vi "#EVENT Main.vi"() -> ()   [LabVIEW 2013]
panel:
  in  "BOOLEAN":bool
  out "COLD STORAGE LOCATIONS":string
  out "LOW MOISTURE":bool
  out "INTERMEDIATE MOISTURE":bool
  out "HIGH MOISTURE":bool
  out "MOISTURE LEVEL(ppm)":dbl
  out "pH VALUE":dbl
  out "SUGGESTED CROP":string
  out "Alert":bool
  out "POSITION":string
  out "Current Latitude [deg]":string
  out "Current Longitude [deg]":string
  in  "USER EMAIL Id":string="pankaj7897@outlook.com"
  out "CURRENT FARM STATUS":T1(plugin-control)
  out "WEATHER FORECAST":T2(array[cluster])
  # "SOIL ANALYSIS REPORT"
  # "SECURITY REPORT"
  # "MOISTURE READINGS"
  # "COLD STORAGE HOUSES NEAR YOU"
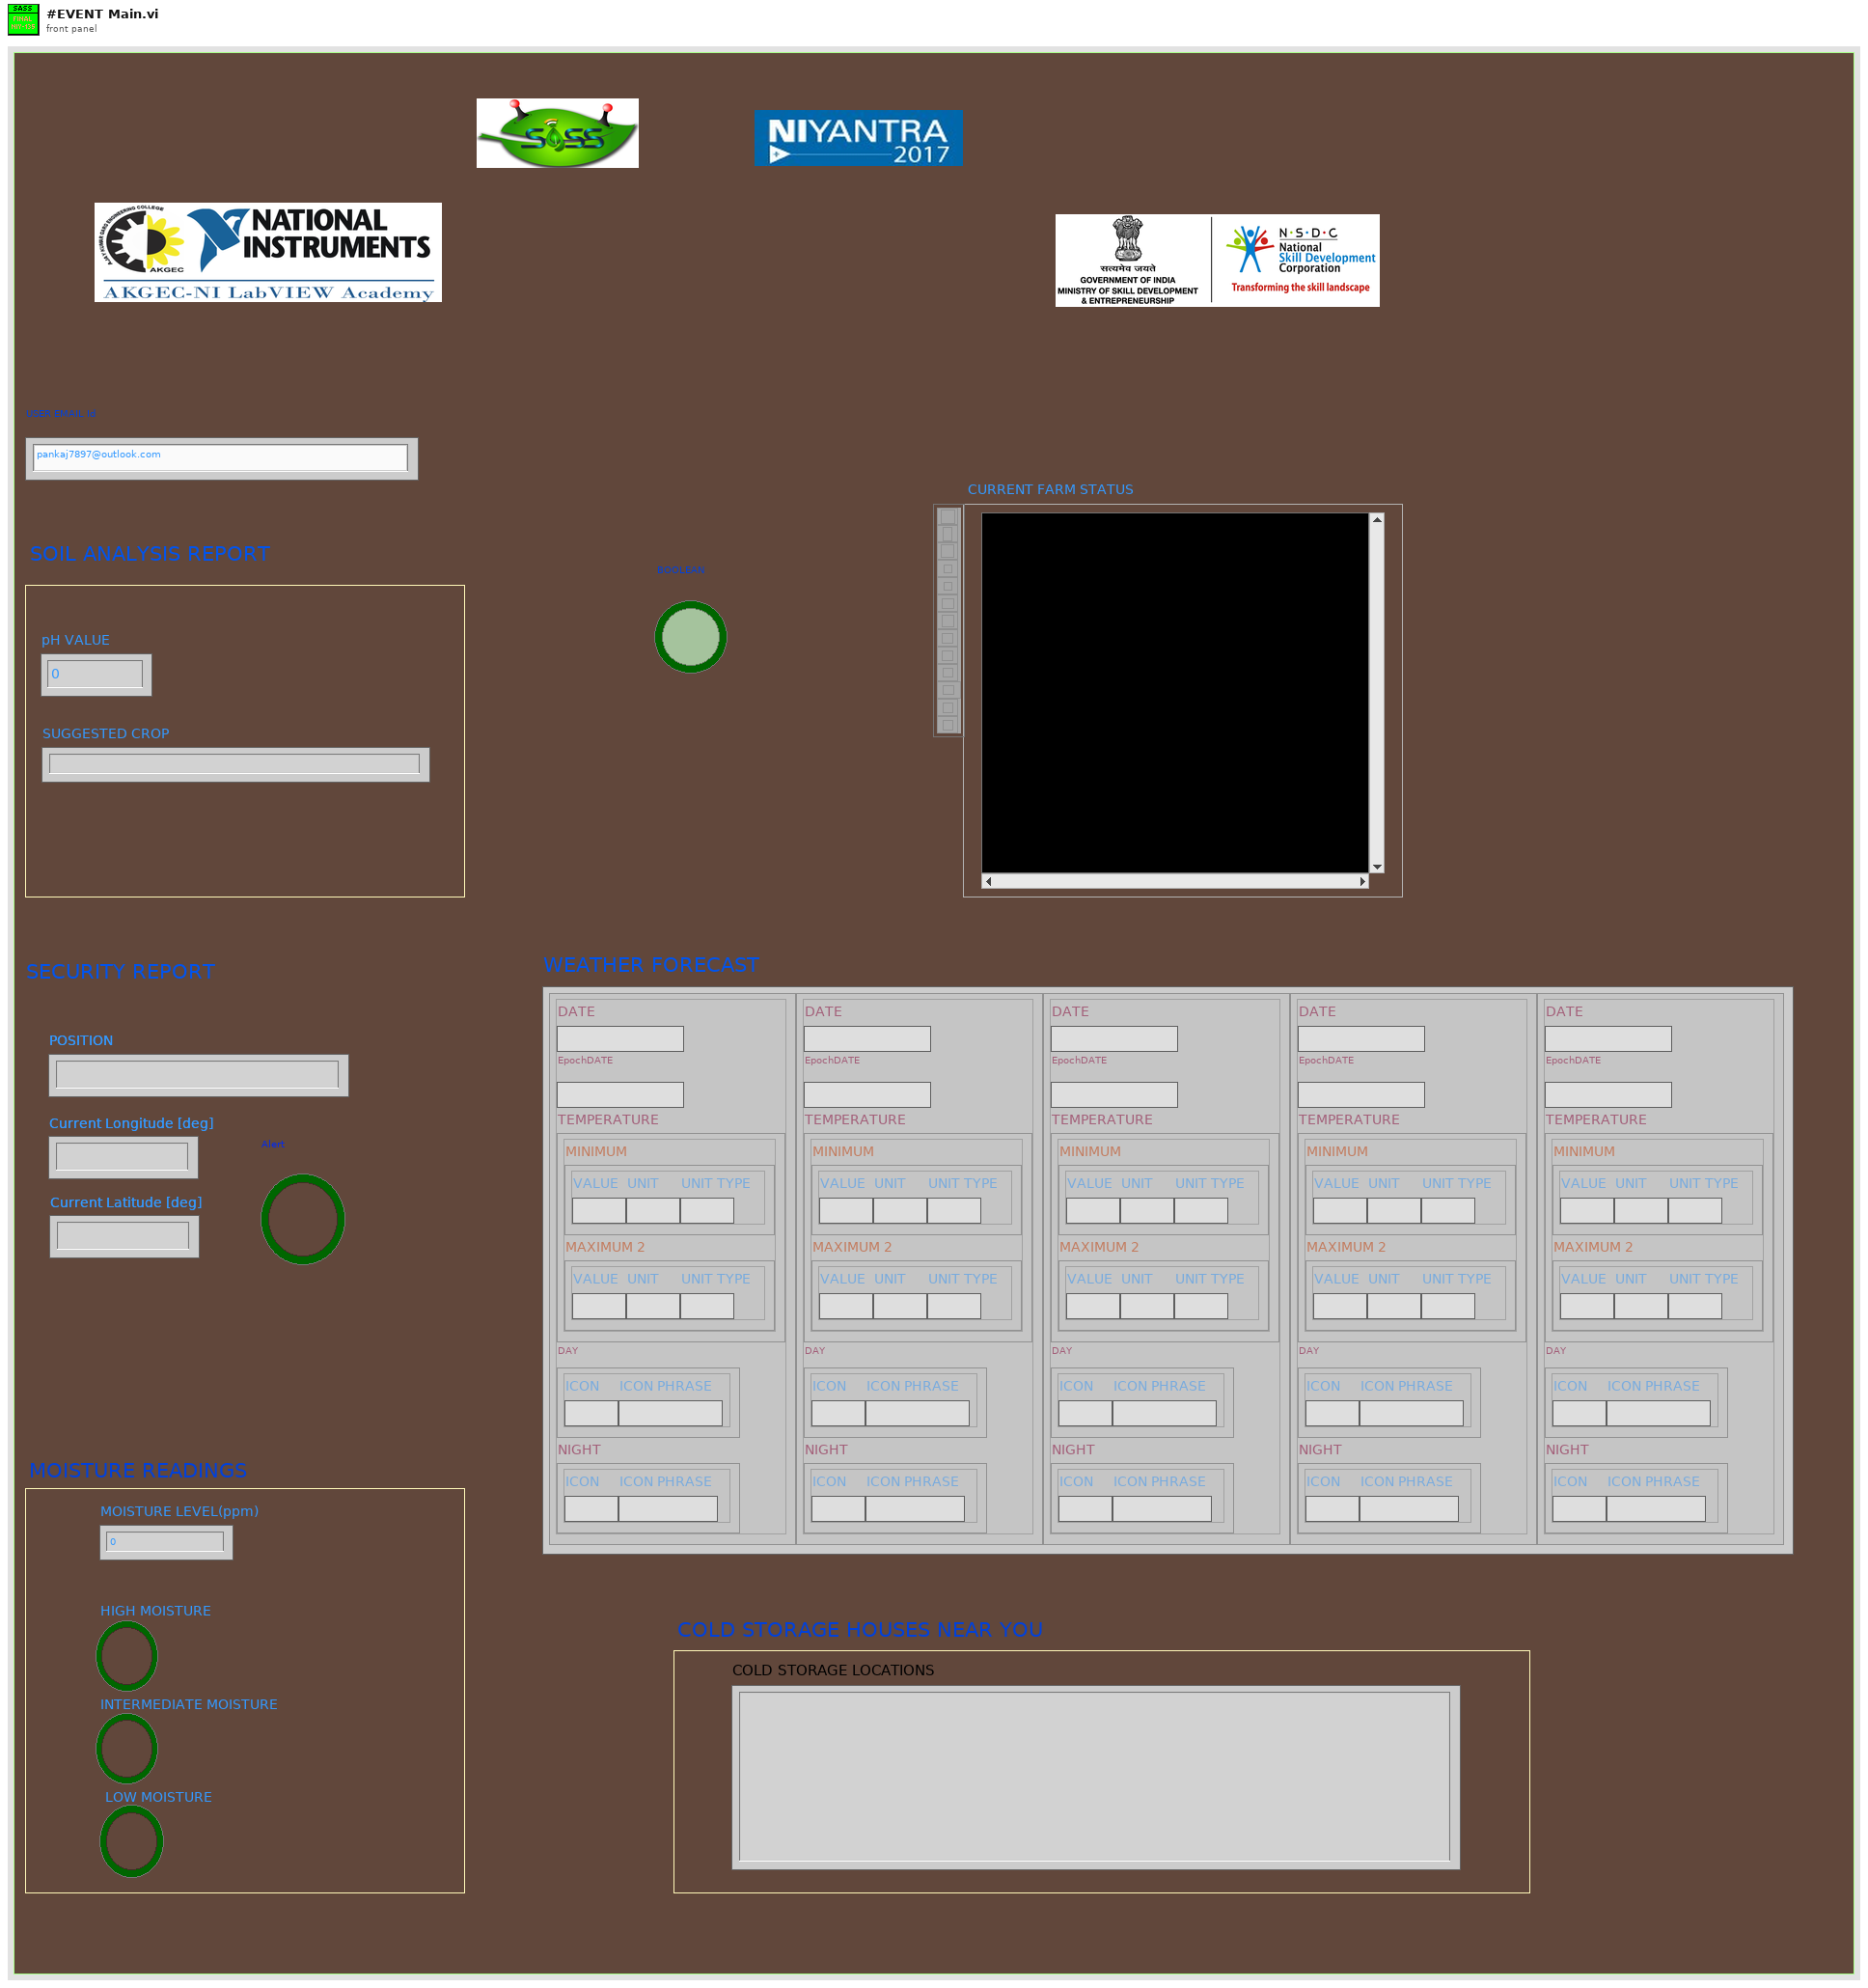
[diagram p1: front panel]
types:
  T1 = typedef "IMAQ Image.ctl" = refnum<image>
  T2 = cluster{"DATE":string, "EpochDATE":string, "TEMPERATURE":cluster{"MINIMUM":cluster{"VALUE":string, "UNIT":string, "UNIT TYPE":string}, "MAXIMUM 2":cluster{"VALUE":string, "UNIT":string, "UNIT TYPE":string}}, "DAY ":cluster{"ICON":string, "ICON PHRASE":string}, "NIGHT":cluster{"ICON":string, "ICON PHRASE":string}}[]
  T3 = cluster{"DATE":string, "EpochDATE":string, "TEMPERATURE":cluster{"MINIMUM":cluster{"VALUE":string, "UNIT":string, "UNIT TYPE 3":string}, "MAXIMUM 2":cluster{"VALUE":string, "UNIT":string, "UNIT TYPE":string}}, "DAY ":cluster{"ICON":string, "ICON PHRASE":string}, "NIGHT":cluster{"ICON":string, "ICON PHRASE":string}}[]
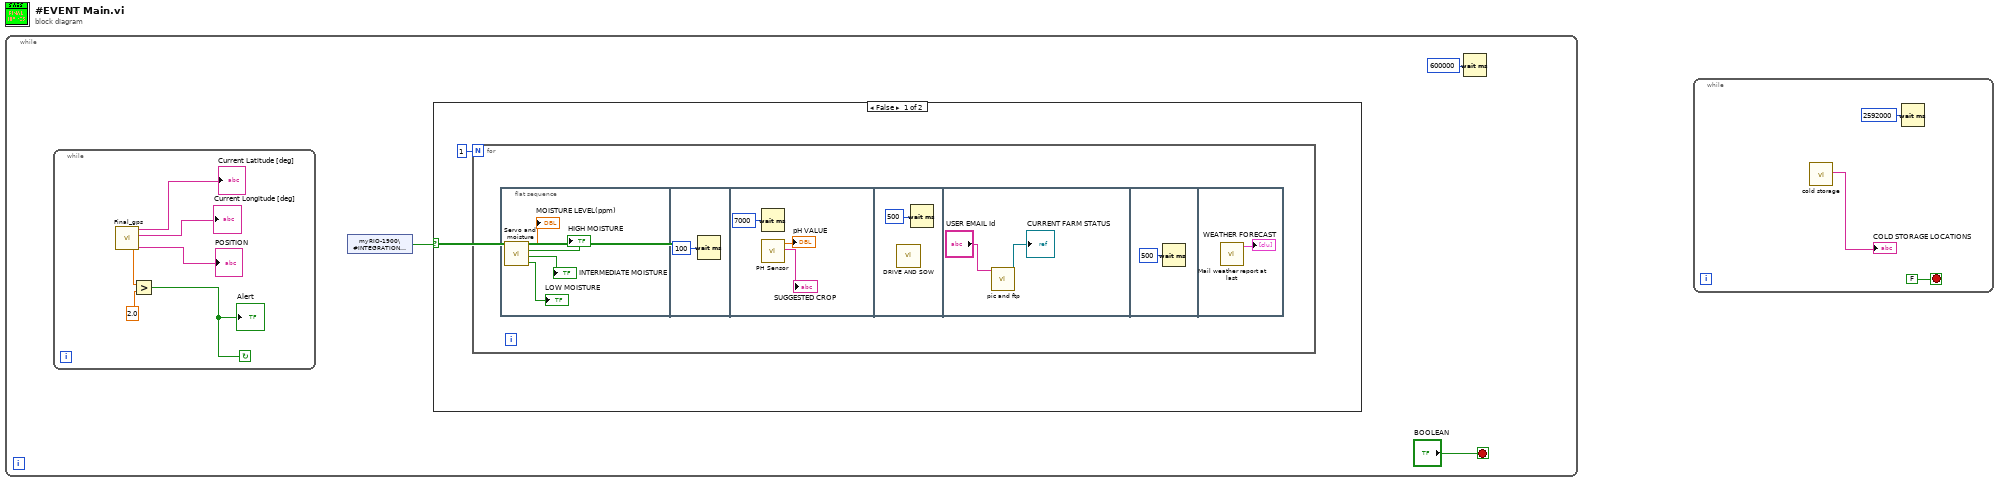
[diagram p0: block diagram]
diagram:
  n1 = while {
    stop <- "BOOLEAN" stop-if-true
    n2 = while {
      stop <- w18 continue-if-true
      n3 = call "Final_gps.vi"() -> ("POSITION"=→"POSITION":string, "Distance to Destination m"=w22:dbl, "Current Longitude [deg]"=→"Current Longitude [deg]":string, "Current Latitude [deg]"=→"Current Latitude [deg]":string)  [unwired: 8 in]
      n4 = Greater?(x=w22, y=2.0) -> (0:w18:bool)
      "Alert" <- w18
    }
    n5 = shared-variable "myRIO-1900\\#INTEGRATION COMPLETE.lvlib\\Variable"() -> (w1:bool)  [unwired: 1 in, 1 out]
    n6 = case shown="False" w1 {
      frame False {
        n7 = for {
          N: 1 -> [_]
          n8 = flat-sequence {
            frame #0 {
              n9 = call "Servo and moisture.vi"() -> ("LOW MOISTURE"=→"LOW MOISTURE":bool, "INTERMEDIATE MOISTURE"=→"INTERMEDIATE MOISTURE":bool, "HIGH MOISTURE"=→"HIGH MOISTURE":bool, "MOISTURE LEVEL(ppm)"=→"MOISTURE LEVEL(ppm)":dbl)  [unwired: 8 in]
            }
            frame #1 {
              n10 = Wait (ms)(milliseconds to wait=u32 100) -> ()  [unwired: 1 out]
            }
            frame #2 {
              n11 = call "PH Sensor.vi"() -> ("SUGGESTED CROP"=→"SUGGESTED CROP":string, "pH VALUE"=→"pH VALUE":dbl)  [unwired: 10 in]
              n12 = Wait (ms)(milliseconds to wait=u32 7000) -> ()  [unwired: 1 out]
            }
            frame #3 {
              n13 = call "DRIVE AND SOW.vi"() -> ()  [unwired: 12 in]
              n14 = Wait (ms)(milliseconds to wait=u32 500) -> ()  [unwired: 1 out]
            }
            frame #4 {
              n15 = call "pic and ftp.vi"("To: 2"="USER EMAIL Id") -> ("Image Out"=→"CURRENT FARM STATUS":T1)  [unwired: 10 in]
            }
            frame #5 {
              n16 = Wait (ms)(milliseconds to wait=u32 500) -> ()  [unwired: 1 out]
            }
            frame #6 {
              n17 = call "Mail weather report at last.vi"() -> ("Array 3"=→"WEATHER FORECAST":T3)  [unwired: 11 in]
            }
          }
        }
      }
      frame True {
      }
    }
    n18 = Wait (ms)(milliseconds to wait=u32 600000) -> ()  [unwired: 1 out]
  }
  n19 = while {
    stop <- FALSE stop-if-true
    n20 = call "cold storage.vi"() -> ("Subject 2"=→"COLD STORAGE LOCATIONS":string)  [unwired: 11 in]
    n21 = Wait (ms)(milliseconds to wait=u32 2592000) -> ()  [unwired: 1 out]
  }
